vi "setUp.vi"(8 "error in (no error)":errorcluster, 11 "reference in":refnum<class "ListImp_Common.lvclass">) -> (0 "error out":errorcluster, 3 "reference out":refnum<class "ListImp_Common.lvclass">)   [LabVIEW 2013, in "ListImp_Common.lvclass"]
doc: "setUp runs prior to the test method during test execution. Use this method to initialize any object data required by your tests."
uses:
  ListImp_Common.lvclass
  <vilib>/addons/_JKI Toolkits/VI Tester/TestCase.llb/TestCase.lvclass
  source/LapDog.Collections.Lists/ListImp/ListImp.lvclass
  source/LapDog.Collections.Common/I32/I32.lvclass
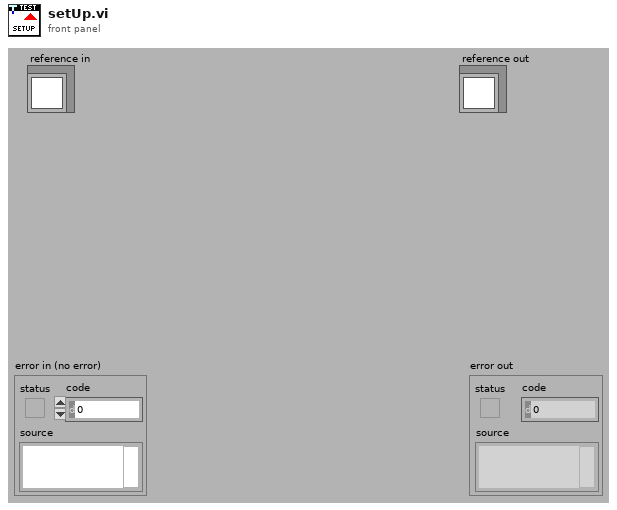
[diagram p1: front panel]
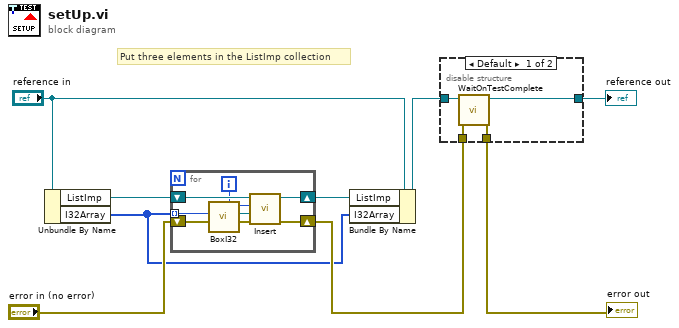
[diagram p0: block diagram]
diagram:
  # "Put three elements in the ListImp collection"
  n1 = Unbundle By Name("reference in") -> ("ListImp"=w2:refnum<class "ListImp.lvclass">, "I32Array"=w1:i32[])
  n2 = for {
    shift-right: [w15] -> w6
    shift-left: w2 -> [w16]
    shift-right: [w13] -> w4
    shift-left: "error in (no error)" -> [w12]
    tunnel: w1 -> [w10] mode=indexing
    i -> [w11]
    n3 = call "BoxI32.vi"("Numeric"=w10) -> ("I32 out"=w14:refnum<class "I32.lvclass">)  [unwired: 10 in]
    n4 = call-dynamic "Insert.vi"("error in (no error)"=w12, "Item"=w14, "Index"=w11, "ListImp in"=w16) -> ("error out"=w13:errorcluster, "ListImp out"=w15:refnum<class "ListImp.lvclass">)  [unwired: 6 in]
  }
  n5 = Bundle By Name(cluster="reference in", "ListImp"=w6, "I32Array"=w1) -> (w7:refnum<class "ListImp_Common.lvclass">)
  n6 = disable-structure shown="Default" {
    disable-tunnel: w4 -> [w20 w21]
    disable-tunnel: [w19 w21] -> w9
    disable-tunnel: [w18 w22] -> w8
    disable-tunnel: w7 -> [w17 w22]
    frame condition #0 (active) {
      n7 = call <vilib>:"WaitOnTestComplete.vi"("error in (no error)"=w20, "TestCase in"=w17) -> ("error out"=w19:errorcluster, "TestCase out"=w18:refnum<class "ListImp_Common.lvclass">)  [unwired: 8 in]
    }
    frame condition #1 {
    }
  }
  "error out" <- w9
  "reference out" <- w8
